vi "Test Customer Pick Up Order Broadcasts State.vi"(8 "error in (no error)":errorcluster, 11 "Customer Test in":refnum<class "Customer Test.lvclass">) -> (0 "error out":errorcluster, 3 "Customer Test out":refnum<class "Customer Test.lvclass">)   [LabVIEW 2020, in "Customer Test.lvclass"]
uses:
  Customer Test.lvclass
  C:/Program Files (x86)/National Instruments/LabVIEW 2020/vi.lib/Astemes/LUnit/Test Case.lvclass
  Processes/People/Customers/Customer/Customer.lvclass
  C:/Program Files (x86)/National Instruments/LabVIEW 2020/vi.lib/Astemes/Triarc Framework/Process/Process.lvclass
  Support/Beverages/Beverage/Beverage.lvclass
  Processes/People/Customers/Customer/Public/Order State.ctl
  <vilib>/Astemes/Triarc Framework/Process/Process.lvclass/Process.ctl
  <vilib>/Astemes/LUnit/Test Case.lvclass/Test Case.ctl
  <vilib>/Astemes/Triarc Framework/Process/Public/Lifecycle/Get Lifecycle State.vi
  <vilib>/Astemes/Triarc Framework/Support/Execution timer.vi
  <vilib>/Astemes/LUnit/Append Fail Result.vi
  <vilib>/Astemes/LUnit/Append Pass Result.vi
  <vilib>/Astemes/Triarc Framework/Process/Private/SubVIs/Wait for finish.vi
  <vilib>/Astemes/Triarc Framework/Process/Private/SubVIs/Set Lifecycle State.vi
  <vilib>/Astemes/Triarc Framework/Process/Protected/Messaging/Send Message.vi
  <vilib>/Utility/error.llb/Clear Errors.vi
  <vilib>/Astemes/Triarc Framework/Process/Private/SubVIs/Handle Debug Data.vi
  <vilib>/Astemes/Triarc Framework/Logging/Log Debug.vi
  <vilib>/AdvancedString/1D String Array to Delimited String.vi
  <vilib>/Utility/High Resolution Relative Seconds.vi
  <vilib>/Utility/error.llb/Error Cluster From Error Code.vi
  <vilib>/Astemes/Triarc Framework/Support/Dequeue Broadcast Message.vi
  <vilib>/Astemes/Triarc Framework/Process/Public/Read Name.vi
  <vilib>/Astemes/Triarc Framework/Callback/Callback.lvclass
  <vilib>/Astemes/Triarc Framework/Process/Process.lvclass
  <vilib>/Astemes/LUnit/Test Case.lvclass
  <vilib>/Astemes/Triarc Framework/Support/Broadcast Event Dequeuers.lvlib
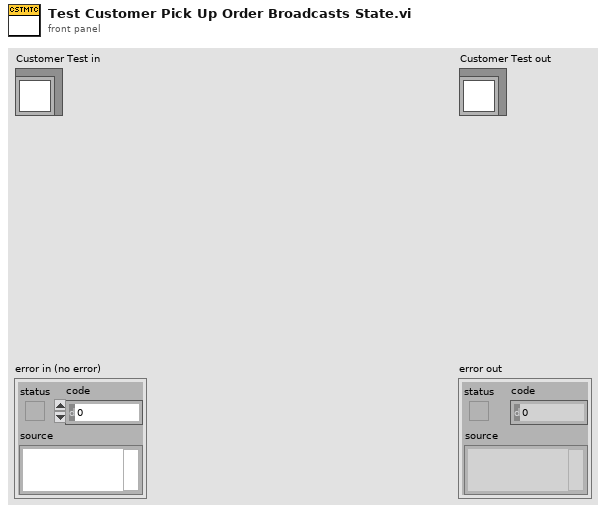
[diagram p1: front panel]
types:
  T1 = typedef "Customer.lvclass/Order State.ctl" = cluster{"Order In Progress?":bool, "Order Number":u32, "Order Price":dbl, "Items Ordered":u32, "Items Received":u32, "Items Picked Up":string}
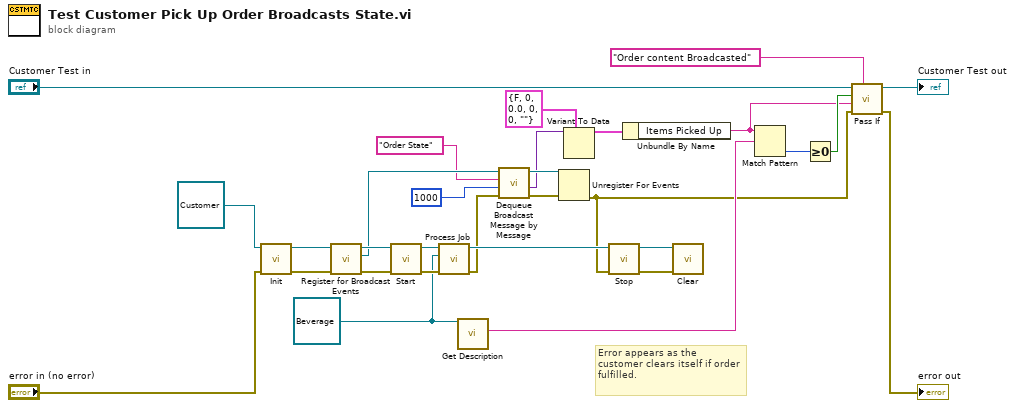
[diagram p0: block diagram]
diagram:
  w9 = refnum<class "Beverage.lvclass"> refnum ("Beverage.lvclass")
  # "Error appears as the customer clears itself if order fulfilled."
  n1 = call-dynamic "Init.vi"("error in (no error)"="error in (no error)", "View In"=refnum<class "Customer.lvclass"> refnum ("Customer.lvclass")) -> ("error out"=w26:errorcluster, "View Out"=w27:refnum<class "Customer.lvclass">)  [unwired: 8 in]
  n2 = call <vilib>:"Register for Broadcast Events.vi"("error in (no error)"=w26, "Process In"=w27) -> ("error out"=w29:errorcluster, "Event Registration Refnum Out"=w23:refnum<event-registration>, "Process Out"=w28:refnum<class "Customer.lvclass">)  [unwired: 7 in]
  n3 = call <vilib>:"Start.vi"("error in (no error)"=w29, "Process In"=w28) -> ("error out"=w20:errorcluster, "Process Out"=w22:refnum<class "Customer.lvclass">)  [unwired: 7 in, 1 out]
  n4 = call-dynamic "Process Job.vi"("error in (no error)"=w20, "Job"=w9, "Process Job In"=w22) -> ("error out"=w19:errorcluster, "Process Job Out"=w21:refnum<class "Customer.lvclass">)  [unwired: 7 in]
  n5 = call "Get Description.vi"("Beverage in"=w9) -> ("Description"=w6:string)  [unwired: 8 in, 2 out]
  n6 = call <vilib>:"Dequeue Broadcast Message by Message.vi"("error in (no error)"=w19, "Timeout (-1)"=1000, "Message"="Order State", "Event Registration Refnum"=w23) -> ("error out"=w18:errorcluster, "Message Data"=w10:variant, "Event Registration Refnum Out"=w13:refnum<event-registration>)  [unwired: 3 in, 2 out]
  n7 = Unregister For Events(event registration refnum=w13, error in=w18) -> (error out=w1:errorcluster)
  n8 = Variant To Data(type=T1 {"Order In Progress?"=FALSE, "Order Number"=0, "Order Price"=0.0, "Items Ordered"=0, "Items Received"=0, "Items Picked Up"=""} ("Order State"), Variant=w10) -> (data=w7:T1)  [unwired: 1 in, 1 out]
  n9 = call <vilib>:"Stop.vi"("error in (no error)"=w1, "Process In"=w21) -> ("error out"=w2:errorcluster, "Process Out"=w25:refnum<class "Customer.lvclass">)  [unwired: 7 in, 1 out]
  n10 = Unbundle By Name(w7) -> ("Items Picked Up"=w3:string)
  n11 = call-dynamic "Clear.vi"("error in (no error)"=w2, "View In"=w25) -> ()  [unwired: 9 in, 1 out]
  n12 = Match Pattern(string=w3, regular expression=w6) -> (offset past match=w5:i32)  [unwired: 1 in, 3 out]
  n13 = Greater Or Equal To 0?(x=w5) -> (x >= 0?=w4:bool)
  n14 = call <vilib>:"Pass If.vi"("Description"="Order content Broadcasted", "error in (no error)"=w1, "Message"=w3, "Pass?"=w4, "LUnit Test Case In"="Customer Test in") -> ("error out"=→"error out":errorcluster, "LUnit Test Case Out"=→"Customer Test out":refnum<class "Customer Test.lvclass">)  [unwired: 5 in]
